vi "Core.vi"(11 "API.lvclass":refnum<class "API.lvclass">) -> (2 "Waveform Chart":i32(graph), 3 "Numeric":i32)   [LabVIEW 2024, in "Data Generator Actor.lvclass"]
uses:
  Data Generator Actor.lvclass
  API/API.lvclass
  Data Generator Actor.lvclass/Data Generator Actor.ctl
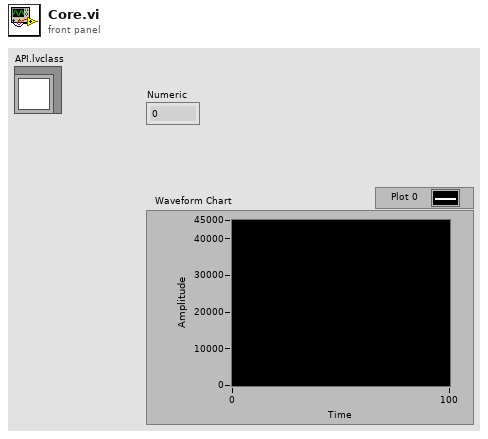
[diagram p1: front panel]
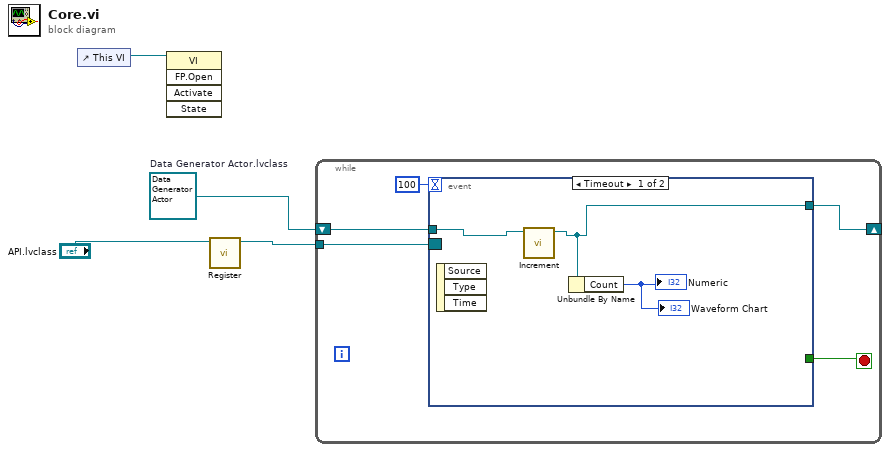
[diagram p0: block diagram]
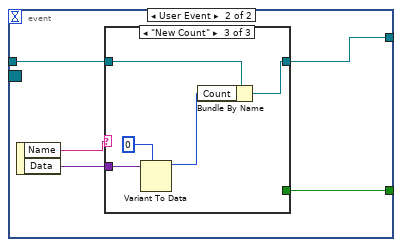
[diagram p2: hidden frame]
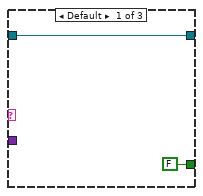
[diagram p3: hidden frame]
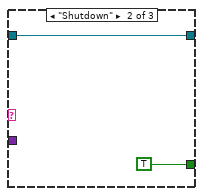
[diagram p4: hidden frame]
diagram:
  w2 = refnum<class "Data Generator Actor.lvclass"> refnum  # Data Generator Actor.lvclass
  n1 = control-ref of="This VI"() -> (w1:refnum<vi>)
  n2 = invoke class="VI" method="FP.Open"(reference=w1) -> ()  [unwired: 4 in, 5 out]
  n3 = call "Register.vi"("API in"="API.lvclass") -> ("Message"=w4:refnum<event-registration>)  [unwired: 10 in]
  n4 = while {
    tunnel: w4 -> [w9]
    shift-right: [w5] -> _
    shift-left: w2 -> [w7]
    stop <- w8 stop-if-true
    n5 = event shown="[0] Timeout" {
      selector: w9 -> [_ _]
      dyn-events: _ -> [_ _]
      timeout: 100 -> [_ _]
      tunnel: [_ w16] -> w8
      tunnel: w7 -> [w12 w14]
      tunnel: [w11 w13] -> w5
      event Timeout {
        n6 = event-data() -> ()  [unwired: 1 in, 3 out]
        n7 = call "Increment.vi"("Data Generator Actor in"=w12) -> ("Data Generator Actor out"=w11:refnum<class "Data Generator Actor.lvclass">)  [unwired: 10 in]
        n8 = Unbundle By Name(w11) -> ("Count"=→"Numeric" →"Waveform Chart":i32)
      }
      event User Event {
        n9 = event-data() -> ("Name"=w17:string, "Data"=w15:variant)  [unwired: 1 in]
        n10 = case shown="\"New Count\"" w17 {
          tunnel: [FALSE TRUE _] -> w16
          tunnel: w15 -> [_ _ w26]
          tunnel: w14 -> [w18 w20 w24]
          tunnel: [w18 w20 w22] -> w13
          frame Default {
          }
          frame "Shutdown" {
          }
          frame "New Count" {
            n11 = Variant To Data(type=0, Variant=w26) -> (data=w23:i32)  [unwired: 1 in, 1 out]
            n12 = Bundle By Name(cluster=w24, "Count"=w23) -> (w22:refnum<class "Data Generator Actor.lvclass">)
          }
        }
      }
    }
  }
